vi "Write Abs_Waveform.lvclass.vi"(8 "error in (no error)":errorcluster, 10 "Abs_Waveform.lvclass":refnum<class "Abs_Waveform.lvclass">, 11 "AbsFunc_Two Term_WFM in":refnum<class "AbsFunc_One Term_WFM_Numeric.lvclass">) -> (0 "error out":errorcluster, 3 "AbsFunc_Two Term_WFM out":refnum<class "AbsFunc_One Term_WFM_Numeric.lvclass">)   [LabVIEW 2021, in "AbsFunc_One Term_WFM_Numeric.lvclass"]
uses:
  AbsFunc_One Term_WFM_Numeric.lvclass
  Abs_Types/Waveform/Abs_Waveform.lvclass
  AbsFunc_One Term_WFM_Numeric.lvclass/AbsFunc_One Term_WFM_Numeric.ctl
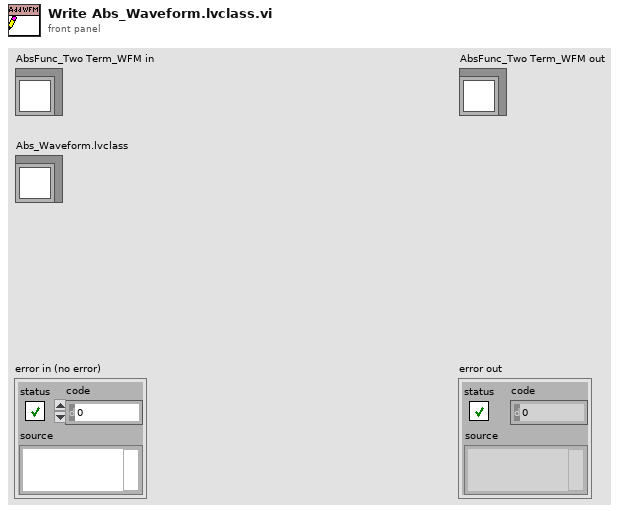
[diagram p1: front panel]
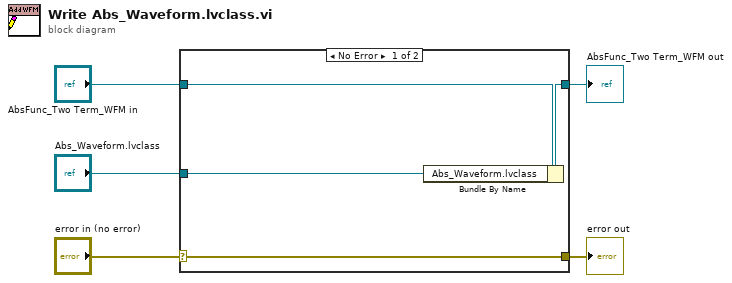
[diagram p0: block diagram]
diagram:
  n1 = case shown="No Error" "error in (no error)" {
    selector: "error in (no error)" -> [w9 w10]
    tunnel: [w9 w10] -> w4
    tunnel: [w7 w11] -> w2
    tunnel: "AbsFunc_Two Term_WFM in" -> [w8 w11]
    tunnel: "Abs_Waveform.lvclass" -> [w6 _]
    frame No Error {
      n2 = Bundle By Name(cluster=w8, "Abs_Waveform.lvclass"=w6) -> (w7:refnum<class "AbsFunc_One Term_WFM_Numeric.lvclass">)
    }
    frame Error {
    }
  }
  "error out" <- w4
  "AbsFunc_Two Term_WFM out" <- w2
